vi "leggi tipo collegamento.vi"(8 "error in (no error)":errorcluster, 9 "lingua":i32, 10 "ID disponibili":string[](array[string])=["3"], 11 "ID":i32) -> (0 "error out":errorcluster, 1 "imp resistomat":T2, 2 "imp resmeter":T3, 3 "ALIMENTAZIONE ELETTRICA":T4, 4 "CALCOLI":T1, 5 "lista":string[](array[string]))   [LabVIEW 2019]
uses:
  TypeDef/Collegamenti_elettrici.ctl
  TypeDef/Control Calcoli.ctl
  Global percorso impostazioni.vi
  <vilib>/Utility/file.llb/Read Delimited Spreadsheet (string).vi
panel:
  out "#rami termica resistomat":i32
  out "#rami freddo resistomat":i32
  out "#rami freddo resmeter":i32
  out "#rami termica resmeter":i32
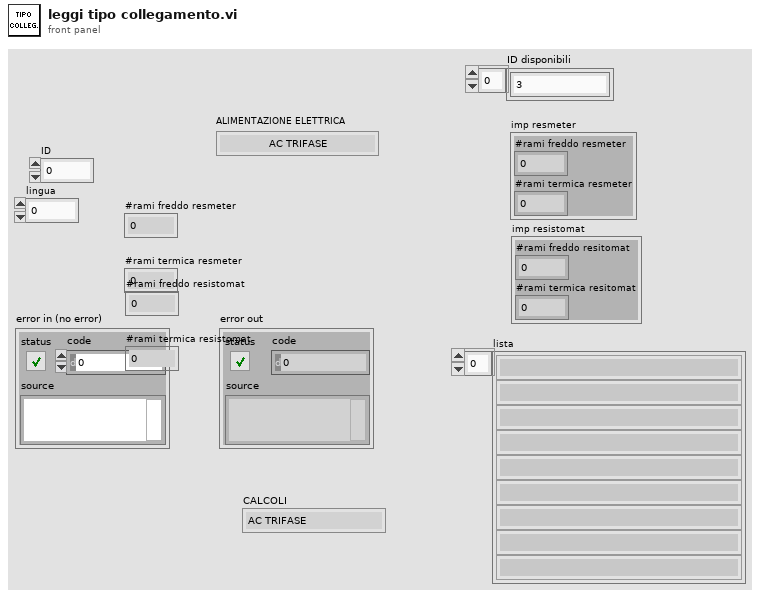
[diagram p1: front panel]
types:
  T1 = typedef "Control Calcoli.ctl" = enum16{"AC TRIFASE", "AC MONOFASE", "DC ECCITAZIONE", "DC NO ECCITAZIONE", "POMPA TRIFASE", "POMPA MONOFASE", "GENERICO", "TRASFORMATORE", "ALTERNATORE TRASCINATO", "GRUPPO ELETTROGENO"}
  T2 = cluster{"#rami freddo resitomat":i32, "#rami termica resitomat":i32}
  T3 = cluster{"#rami freddo resmeter":i32, "#rami termica resmeter":i32}
  T4 = typedef "Collegamenti_elettrici.ctl" = enum16{"AC TRIFASE", "AC TRIFASE + FRENO", "AC MONOFASE", "DC CON ECCITAZIONE", "DC CON ECCITAZIONE + FRENO", "DC NO ECCITAZIONE", "DC NO ECCITAZIONE + FRENO", "FRENO TRASC + AFE", "SOLO FRENO", "CARICO RESISTIVO", "GENERICO", "SOLO ACQUISITORE", "SCORTA 4", "SCORTA 5", "SCORTA 6"}
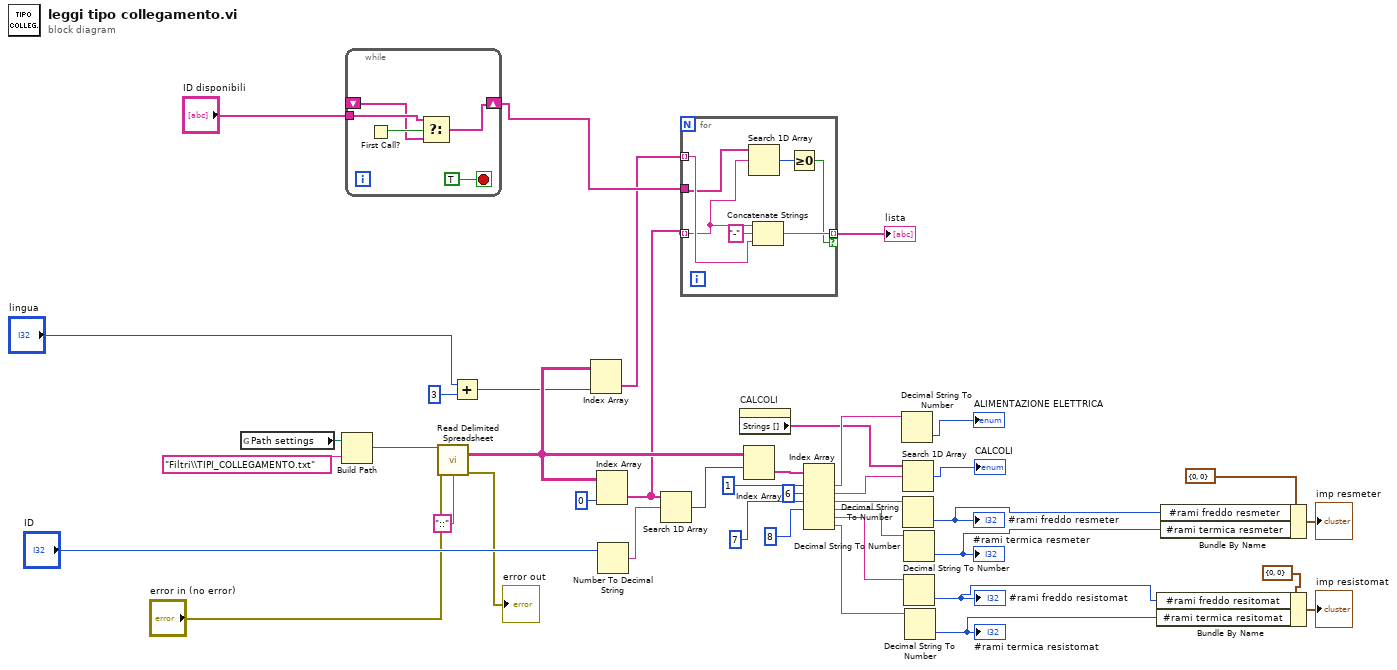
[diagram p0: block diagram]
diagram:
  n1 = global read "Global percorso impostazioni.vi" "Path settings"() -> (w30:path)
  n2 = Build Path(base path=w30, name or relative path="Filtri\\TIPI_COLLEGAMENTO.txt") -> (appended path=w32:path)
  n3 = while {
    shift-right: [w44] -> w5
    shift-left: _ -> [w43]
    tunnel: "ID disponibili" -> [w45]
    stop <- TRUE stop-if-true
    n4 = First Call?() -> (First Call?: T/F=w46:bool)
    n5 = Select(t=w45, s=w46, f=w43) -> (s? t:f=w44:string[])
  }
  n6 = call-poly <vilib>:"Read Delimited Spreadsheet.vi"("file path (dialog if empty)"=w32, "error in (no error)"="error in (no error)", "delimiter (\\t)"="::") -> ("all rows"=w27:string[][], "error out"=→"error out":errorcluster)  [unwired: 7 in, 4 out]
  n7 = Add(x="lingua", y=3) -> (x+y=w24:i32)
  n8 = Index Array(array=w27, index (col)=w24) -> (element=w2:string[])  [unwired: 1 in]
  n9 = Index Array(array=w27, index (col)=0 ("disabled index (col)")) -> (element=w3:string[])  [unwired: 1 in]
  n10 = Number To Decimal String(number="ID") -> (decimal integer string=w35:string)  [unwired: 1 in]
  n11 = Search 1D Array(1D array=w3, element=w35) -> (index of element=w36:i32)  [unwired: 1 in]
  n12 = for {
    tunnel: w2 -> [w51] mode=indexing
    tunnel: w3 -> [w49] mode=indexing
    tunnel: [w53] -> w1 mode=indexing if=w48
    tunnel: w5 -> [w50]
    n13 = Search 1D Array(1D array=w50, element=w49) -> (index of element=w47:i32)  [unwired: 1 in]
    n14 = Concatenate Strings(w49, "-" ("string"), w51) -> (w53:string)
    n15 = Greater Or Equal To 0?(x=w47) -> (x >= 0?=w48:bool)
  }
  "lista" <- w1
  n16 = property on="CALCOLI" class="Enum (strict)"() -> ("Strings []"=w8:string[])  [unwired: 2 in, 2 out]
  n17 = Index Array(array=w27, index (row)=w36) -> (element=w37:string[])  [unwired: 1 in]
  n18 = Index Array(array=w37, index #1=1 ("index"), index #2=6 ("index"), index #3=7 ("index"), index #4=8 ("index")) -> (element #1=w10:string, element #2=w7:string, element #3=w40:string, element #4=w41:string, element #5=w21:string, element #6=w20:string)  [unwired: 2 in]
  n19 = Decimal String To Number(string=w10) -> (number=→"ALIMENTAZIONE ELETTRICA":i32)  [unwired: 2 in, 1 out]
  n20 = Search 1D Array(1D array=w8, element=w7) -> (index of element=→"CALCOLI":i32)  [unwired: 1 in]
  n21 = Decimal String To Number(string=w40) -> (number=w17:i32)  [unwired: 2 in, 1 out]
  "#rami freddo resmeter" <- w17
  n22 = Decimal String To Number(string=w41) -> (number=w16:i32)  [unwired: 2 in, 1 out]
  "#rami termica resmeter" <- w16
  n23 = Decimal String To Number(string=w21) -> (number=w15:i32)  [unwired: 2 in, 1 out]
  "#rami freddo resistomat" <- w15
  n24 = Decimal String To Number(string=w20) -> (number=w14:i32)  [unwired: 2 in, 1 out]
  "#rami termica resistomat" <- w14
  n25 = Bundle By Name(cluster=T2 {"#rami freddo resitomat"=0, "#rami termica resitomat"=0} ("output cluster"), "#rami freddo resitomat"=w15, "#rami termica resitomat"=w14) -> (→"imp resistomat":T2)
  n26 = Bundle By Name(cluster=T3 {"#rami freddo resmeter"=0, "#rami termica resmeter"=0} ("output cluster"), "#rami freddo resmeter"=w17, "#rami termica resmeter"=w16) -> (→"imp resmeter":T3)
